vi "StreamEngine.Main.Stream.Start.vi"(7 "Stream.Qs.SubProcesses":T1, 8 "error in (no error)":errorcluster, 11 "Parameters":variant) -> (0 "error out":errorcluster, 2 "Stream Ref":T2, 3 "gRPC ID out":T2)   [LabVIEW 2025, in "XNET Bus Monitor Client.lvlib"]
uses:
  XNET Bus Monitor Client.lvlib
  xnet_can_bus_monitor_api_client/xnet_can_bus_monitor_api_client.lvlib
  <vilib>/gRPC/LabVIEW gRPC Library/Shared/grpcId.ctl
  <vilib>/gRPC/LabVIEW gRPC Library/grpc-lvsupport-release.lvlib
  Types/StreamEngine.CmdQueueData.InitialSettings.ctl
  Types/SubProcessEngine.CmdQueueData.Cmd.ctl
  Types/SubProcessEngine.CmdQueueData.ctl
  Types/SubProcessEngine.QueueRefs.ctl
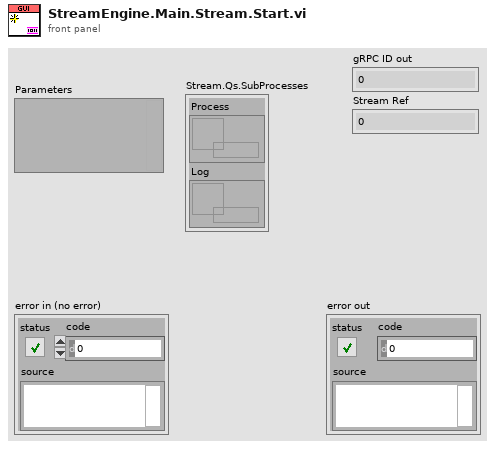
[diagram p1: front panel]
types:
  T1 = typedef "XNET Bus Monitor Client.lvlib/SubProcessEngine.QueueRefs.ctl" = cluster{"Process":refnum<queue>, "Log":refnum<queue>}
  T2 = typedef "grpc-lvsupport-release.lvlib/grpcId.ctl" = u64
  T3 = typedef "XNET Bus Monitor Client.lvlib/StreamEngine.CmdQueueData.InitialSettings.ctl" = cluster{"gRPC ID":T2, "Addon":string, "Project Folder":path}
  T4 = typedef "XNET Bus Monitor Client.lvlib/SubProcessEngine.CmdQueueData.ctl" = cluster{"Cmd":T5, "Parameters":variant}
  T5 = typedef "XNET Bus Monitor Client.lvlib/SubProcessEngine.CmdQueueData.Cmd.ctl" = enum16{"Arm", "Publish", "Stop", "Exit"}
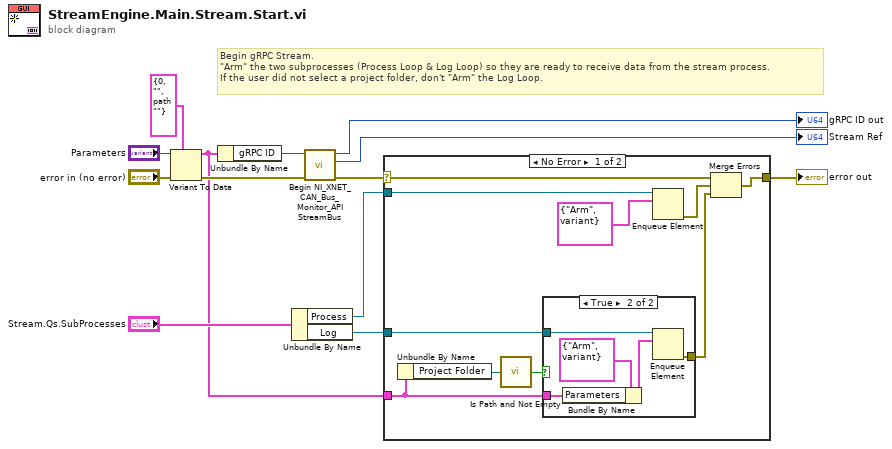
[diagram p0: block diagram]
diagram:
  # "Begin gRPC Stream.\n\"Arm\" the two subprocesses (Process Loop & Log Loop) so they are ready to receive data from the stream process.\nIf the user did not select a project folder, don't \"Arm\" the Log Loop."
  n1 = Variant To Data(error in="error in (no error)", type=T3 {"gRPC ID"=0, "Addon"="", "Project Folder"=path ""} ("cluster"), Variant="Parameters") -> (data=w1:T3, error out=w7:errorcluster)
  n2 = Unbundle By Name(w1) -> ("gRPC ID"=w9:T2)
  n3 = Unbundle By Name("Stream.Qs.SubProcesses") -> ("Process"=w3:refnum<queue>, "Log"=w2:refnum<queue>)
  n4 = call "Begin NI_XNET_CAN_Bus_Monitor_API StreamBus.vi"("error in"=w7, "gRPC ID"=w9) -> ("error out"=w6:errorcluster, "Call Id Out"=→"Stream Ref":T2, "gRPC ID out"=→"gRPC ID out":T2)  [unwired: 7 in]
  n5 = case shown="No Error" w6 {
    selector: w6 -> [w23 w29]
    tunnel: [w19 w29] -> w5
    tunnel: w3 -> [w22 _]
    tunnel: w2 -> [w21 _]
    tunnel: w1 -> [w16 _]
    frame No Error {
      n6 = Unbundle By Name(w16) -> ("Project Folder"=w15:path)
      n7 = call <vilib>:"Is Path and Not Empty.vi"("path"=w15) -> ("Is Path and Not Empty?"=w14:bool)  [unwired: 4 in]
      n8 = case shown="True" w14 {
        tunnel: w21 -> [_ w28]
        tunnel: [_ w26] -> w17
        tunnel: w16 -> [_ w25]
        frame False {
        }
        frame True {
          n9 = Bundle By Name(cluster=T4 {"Cmd"=enum."Arm", "Parameters"=variant} ("element"), "Parameters"=w25) -> (w27:T4)
          n10 = Enqueue Element(queue=w28, element=w27) -> (error out=w26:errorcluster)  [unwired: 2 in, 2 out]
        }
      }
      n11 = Enqueue Element(queue=w22, element=T4 {"Cmd"=enum."Arm", "Parameters"=variant}) -> (error out=w18:errorcluster)  [unwired: 2 in, 2 out]
      n12 = Merge Errors(w23, w18, w17) -> (w19:errorcluster)
    }
    frame Error {
    }
  }
  "error out" <- w5
